vi "Print Interaction.vi"(8 "error in (no error)":errorcluster, 9 "Range":cluster{"Upper":dbl, "Lower":dbl}, 10 "Interaction Type":string, 11 "Abstract Topas in":refnum<class "Abstract Topas.lvclass">) -> (0 "error out":errorcluster, 2 "Interaction Print":string, 3 "Abstract Topas out":refnum<class "Abstract Topas.lvclass">)   [LabVIEW 2020, in "Abstract Topas.lvclass"]
uses:
  Abstract Topas.lvclass
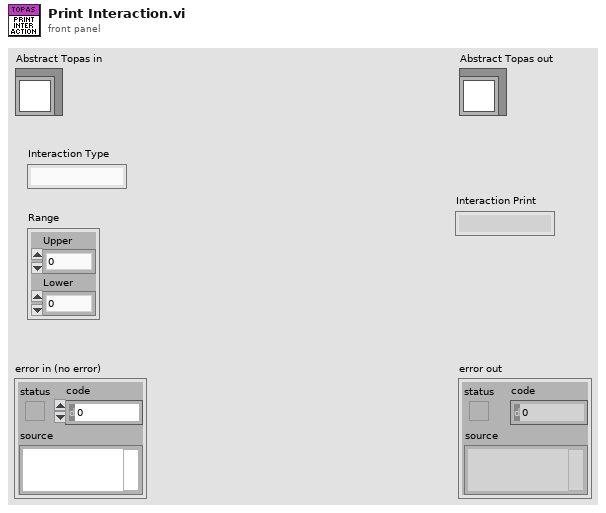
[diagram p1: front panel]
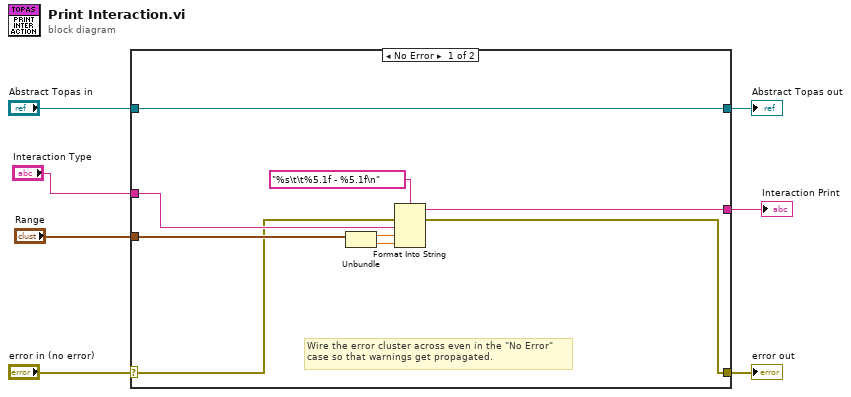
[diagram p0: block diagram]
diagram:
  n1 = case shown="No Error" "error in (no error)" {
    selector: "error in (no error)" -> [w9 w18]
    tunnel: [w8 w18] -> w6
    tunnel: [w16 w17] -> w4
    tunnel: "Abstract Topas in" -> [w16 w17]
    tunnel: "Range" -> [w14 _]
    tunnel: "Interaction Type" -> [w11 _]
    tunnel: [w10 _] -> w1
    frame No Error {
      # "Wire the error cluster across even in the \"No Error\"\ncase so that warnings get propagated."
      n2 = Unbundle(w14) -> ("Upper"=w12:dbl, "Lower"=w13:dbl)
      n3 = Format Into String(format string="%s\t\t%5.1f - %5.1f\n", error in=w9, w11, w12, w13) -> (resulting string=w10:string, error out=w8:errorcluster)  [unwired: 1 in]
    }
    frame Error {
    }
  }
  "error out" <- w6
  "Abstract Topas out" <- w4
  "Interaction Print" <- w1
